vi "TestMoveLine.vi"() -> ()   [LabVIEW 2021, in "Picture2D.lvlib"]
uses:
  Picture2D/Picture2D.lvlib
  PointSpecialized/PointSpecialized.lvclass
  Color/Color.lvclass
  Pen/Pen.lvclass
  Line/Line.lvclass
  C:/Users/Dany/OneDrive/LabVIEW/Class/Picture2D/Point1/Point.lvclass
  C:/Users/Dany/OneDrive/LabVIEW/Class/Picture2D/IDrawable/IDrawable.lvclass
  C:/Users/Dany/OneDrive/LabVIEW/Class/Picture2D/IMovable/IMovable.lvclass
  C:/Users/Dany/OneDrive/LabVIEW/Class/Picture2D/IRotatable/IRotatable.lvclass
  C:/Users/Dany/OneDrive/LabVIEW/Class/Picture2D/IScalable/IScalable.lvclass
  C:/Users/Dany/OneDrive/LabVIEW/Class/Picture2D/Point/PointSpecialized.lvclass
panel:
  in  "Point:EndPoint":cluster{"x":i16, "y":i16}={"x"=-10, "y"=-10}
  in  "Point:StartPoint":cluster{"x":i16, "y":i16}={"x"=-10, "y"=-10}
  in  "Point:ToMove":cluster{"x":i16, "y":i16}={"x"=-10, "y"=-10}
  in  "Pen:Style":T1(ring)
  in  "Pen:Width":u16=10
  in  "Absolute":bool
  out "2D Picture":picture
  in  "Color Box":u32(colorbox)=16711680
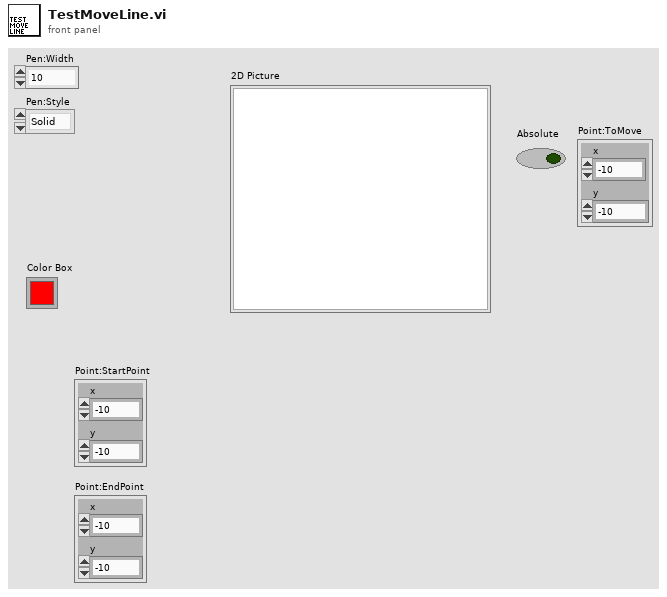
[diagram p1: front panel]
types:
  T1 = enum32{"Solid", "Dash", "Dot", "DashDot", "DashDotDot"}
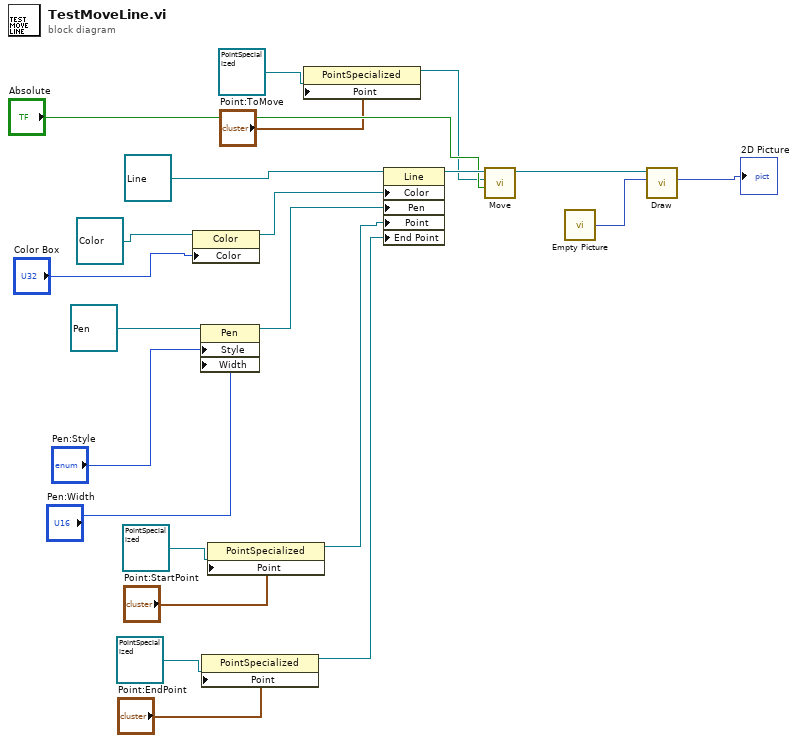
[diagram p0: block diagram]
diagram:
  n1 = property class="Color"(reference=refnum<class "Color.lvclass"> refnum ("Color"), "Color"="Color Box") -> (reference out=w21:refnum<class "Color.lvclass">)  [unwired: 1 in, 1 out]
  n2 = property class="Pen"(reference=refnum<class "Pen.lvclass"> refnum ("Pen"), "Style"="Pen:Style", "Width"="Pen:Width") -> (reference out=w17:refnum<class "Pen.lvclass">)  [unwired: 1 in, 1 out]
  n3 = property class="PointSpecialized"(reference=refnum<class "PointSpecialized.lvclass"> refnum ("Point"), "Point"="Point:EndPoint") -> (reference out=w1:refnum<class "PointSpecialized.lvclass">)  [unwired: 1 in, 1 out]
  n4 = property class="PointSpecialized"(reference=refnum<class "PointSpecialized.lvclass"> refnum ("Point"), "Point"="Point:StartPoint") -> (reference out=w4:refnum<class "PointSpecialized.lvclass">)  [unwired: 1 in, 1 out]
  n5 = property class="PointSpecialized"(reference=refnum<class "PointSpecialized.lvclass"> refnum ("Point"), "Point"="Point:ToMove") -> (reference out=w8:refnum<class "PointSpecialized.lvclass">)  [unwired: 1 in, 1 out]
  n6 = property class="Line"(reference=refnum<class "Line.lvclass"> refnum ("Line"), "Color"=w21, "Pen"=w17, "Point"=w4, "End Point"=w1) -> (reference out=w12:refnum<class "Line.lvclass">)  [unwired: 1 in, 1 out]
  n7 = call-dynamic "Move.vi"("Absolute (T)"="Absolute", "Point"=w8, "Line in"=w12) -> ("Line out"=w11:refnum<class "Line.lvclass">)  [unwired: 7 in, 1 out]
  n8 = call "Empty Picture"() -> ("empty picture"=w14:picture)
  n9 = call-dynamic "Draw.vi"("2D Picture in"=w14, "Line in"=w11) -> ("2D Picture out"=→"2D Picture":picture)  [unwired: 7 in, 2 out]
